vi "testErrorMessageContainsCaller.vi"() -> ()   [LabVIEW 2017, in "Error.Tests.lvlib" / "ExpectationFailedError.lvlib"]
uses:
  ExpectationFailedError.lvlib
  e7830799-5cfa-4e9e-866b-4fb00a76812c.vi
  src/Transparent Assertions/Constraints/IsEqual/Create.vi
  src/Transparent Assertions/Constraints/IsEqual/IsEqual.lvclass
  src/Transparent Assertions/Error/Error.lvlib
panel:
  out "error out":errorcluster
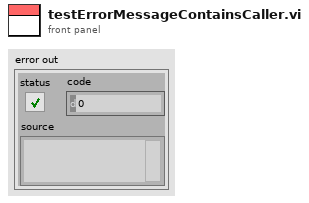
[diagram p1: front panel]
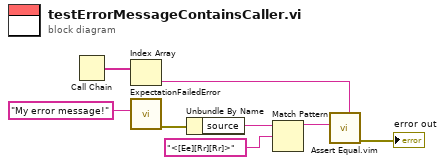
[diagram p0: block diagram]
diagram:
  n1 = Call Chain() -> (call chain=w7:string[])
  n2 = Index Array(array=w7) -> (element=w1:string)  [unwired: 1 in]
  n3 = call "ExpectationFailedError.vi"("Message"="My error message!") -> ("error out"=w5:errorcluster)  [unwired: 10 in]
  n4 = Unbundle By Name(w5) -> ("source"=w4:string)
  n5 = Match Pattern(string=w4, regular expression="<[Ee][Rr][Rr]>") -> (before substring=w2:string)  [unwired: 1 in, 3 out]
  n6 = call "Assert Equal.vim"("Expected"=w1, "Actual"=w2) -> ("error out"=→"error out":errorcluster)  [unwired: 9 in]
